vi "StudentScope - Format Cursor Values.vi"(6 "C2 Voltage In":dbl format="%.3f", 7 "dT In":dbl format="%.3f", 9 "dV In":dbl format="%.3f", 10 "C1 Voltage In":dbl format="%.3f") -> (1 "dV":string, 2 "C1 Voltage":string, 4 "C2 Voltage":string, 5 "dT":string)   [LabVIEW 2015]
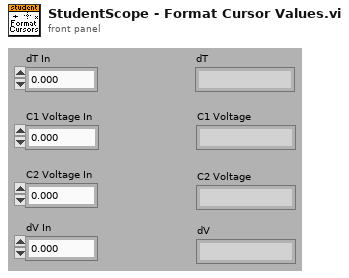
[diagram p1: front panel]
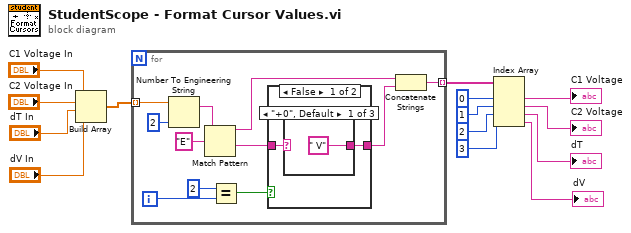
[diagram p0: block diagram]
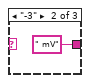
[diagram p2: hidden frame]
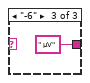
[diagram p3: hidden frame]
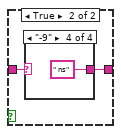
[diagram p4: hidden frame]
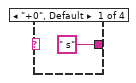
[diagram p5: hidden frame]
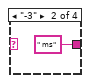
[diagram p6: hidden frame]
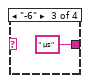
[diagram p7: hidden frame]
diagram:
  n1 = Build Array("C1 Voltage In", "C2 Voltage In", "dT In", "dV In") -> (w12:dbl[])
  n2 = for {
    tunnel: w12 -> [w21] mode=indexing
    tunnel: [w18] -> w11 mode=indexing
    i -> [w16]
    n3 = Number To Engineering String(2:i16 2 ("precision (6)"), 4:w21) -> (0:w25:string)  [unwired: 2 in]
    n4 = Match Pattern(string=w25, regular expression="E" ("string")) -> (before substring=w20:string, after substring=w22:string)  [unwired: 1 in, 2 out]
    n5 = Equal?(x=2, y=w16) -> (x = y?=w17:bool)
    n6 = case shown="False" w17 {
      tunnel: w22 -> [w27 w31]
      tunnel: [w26 w32] -> w19
      frame False {
        n7 = case shown="\"+0\", Default" w27 {
          tunnel: [" V" ("string") " mV" ("string") " µV" ("string")] -> w26
          frame "+0", Default {
          }
          frame "-3" {
          }
          frame "-6" {
          }
        }
      }
      frame True {
        n8 = case shown="\"-9\"" w31 {
          tunnel: [" s" ("string") " ms" ("string") " µs" ("string") " ns" ("string")] -> w32
          frame "+0", Default {
          }
          frame "-3" {
          }
          frame "-6" {
          }
          frame "-9" {
          }
        }
      }
    }
    n9 = Concatenate Strings(w20, w19) -> (w18:string)
  }
  n10 = Index Array(array=w11, index #1=0 ("index"), index #2=1 ("index"), index #3=2 ("index"), index #4=3 ("index")) -> (element #1=→"C1 Voltage":string, element #2=→"C2 Voltage":string, element #3=→"dT":string, element #4=→"dV":string)
